vi "Measurement UI.vi"() -> ()   [LabVIEW 2025]
panel:
  in  "MeasGraphs":T1(tab)
  out "EfficiencyGraph":T2(graph)
  out "LoadRegulationGraph(V/A)":T2(graph)
  out "LoadRegulationGraph(%)":T2(graph)
  out "Load voltage deviation":dbl
  out "Load voltages":dbl
  out "Efficiency":dbl
  out "Load currents":dbl
  in  "Source Voltage":dbl=6.0 format="%#_6pV"
  in  "Load Current":dbl=5.0 format="%#_6pA"
  in  "Buffer graph":bool=TRUE
  in  "Load sense":i32(ring)=1009 caption="SENSE" items=["Local"=1008, "Remote"=1009]
  in  "Source sense":i32(ring)=1009 caption="SENSE" items=["Local"=1008, "Remote"=1009]
  out "Status":string
  in  "Load resource name":refnum<k15> caption="RESOURCE NAME"
  in  "Source resource name":refnum<k15> caption="RESOURCE NAME"
  in  "DUT setup time":dbl=1.0 caption="DUT SETUP TIME" format="%#_6ps"
  in  "Aperture time":dbl=0.005 caption="APERTURE TIME" format="%#_6ps"
  in  "Source delay":dbl=0.005 caption="SOURCE DELAY" format="%#_6ps"
  in  "Load voltage limit range":dbl=6.0 caption="VOLTAGE LIMIT RANGE" format="%#_6pV"
  in  "Source current limit":dbl=25.0 caption="CURRENT LIMIT" format="%#_6pA"
  in  "Source maximum power":dbl=140.0 caption="MAXIMUM POWER" format="%#_6pW"
  in  "Load configuration":string="Load configuration"
  in  "Source configuration":string="Source configuration"
  in  "Measurement settings":string="Measurement settings"
  in  "Nominal output voltage":dbl=3.3 caption="NOMINAL OUTPUT VOLTAGE" format="%#_6pV"
  in  "Mode of operation":T3(ring)=enum."Perform measurement" caption="MODE OF OPERATION"
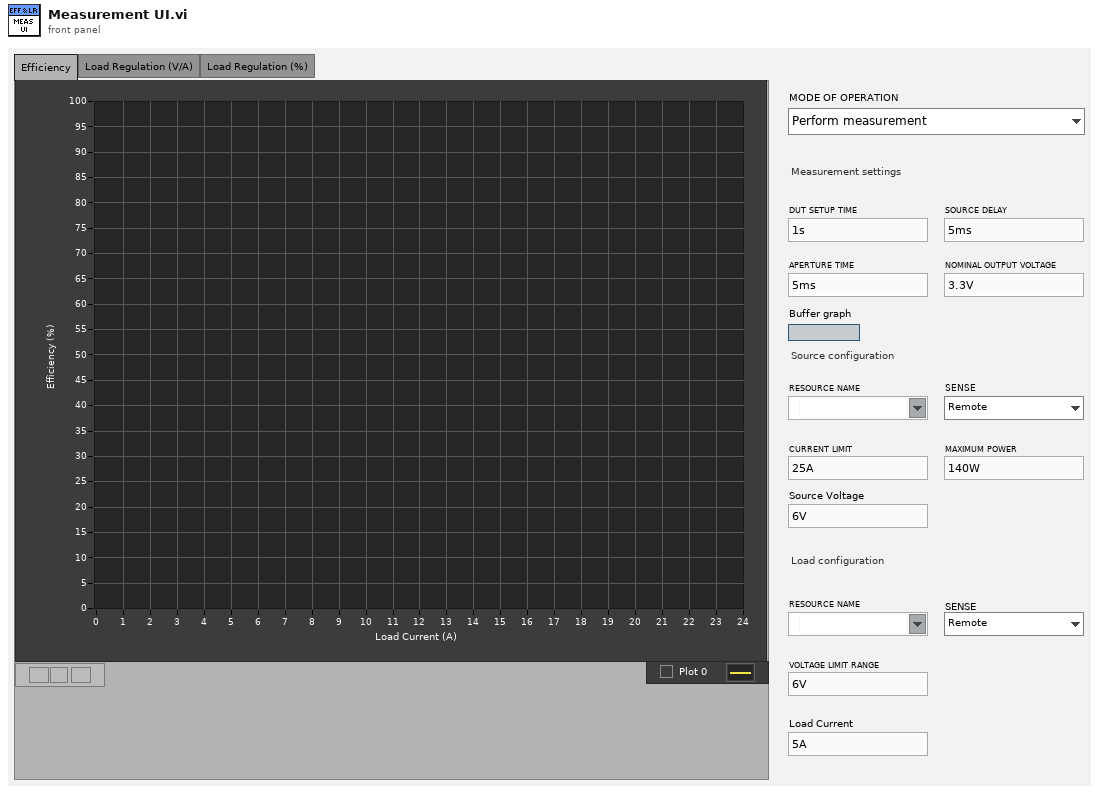
[diagram p1: front panel]
types:
  T1 = enum32{"Efficiency", "Load Regulation (V/A)", "Load Regulation (%)", "Hidden Controls"}
  T2 = cluster{"Load currents":dbl[], "Efficiency":dbl[]}[]
  T3 = enum32{"Power on the DUT", "Perform measurement", "Power off the DUT"}
  T4 = cluster{"Source Voltage[]":dbl[], "Load Current[]":dbl[], "EfficiencyGraph":cluster{"Load currents":dbl[], "Efficiency":dbl[]}[], "LoadGraph(V/A)":cluster{"Load currents":dbl[], "Efficiency":dbl[]}[], "LoadGraph(%)":cluster{"Load currents":dbl[], "Efficiency":dbl[]}[], "Execution Time":timestamp, "Debug file":path}
  T5 = cluster{"Load currents":dbl[], "Efficiency":dbl[]}
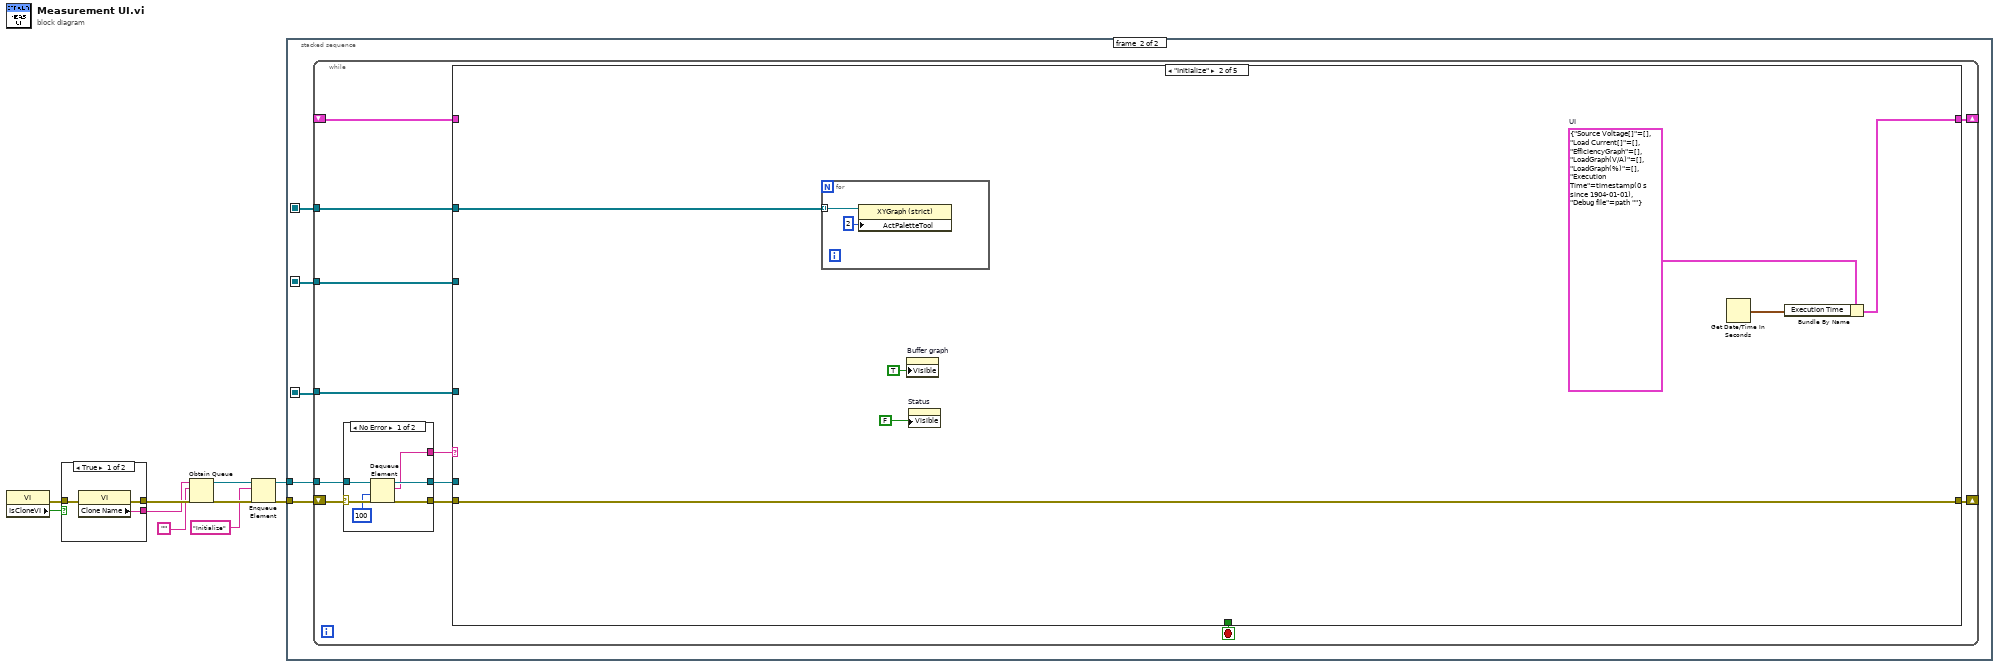
[diagram p0: block diagram]
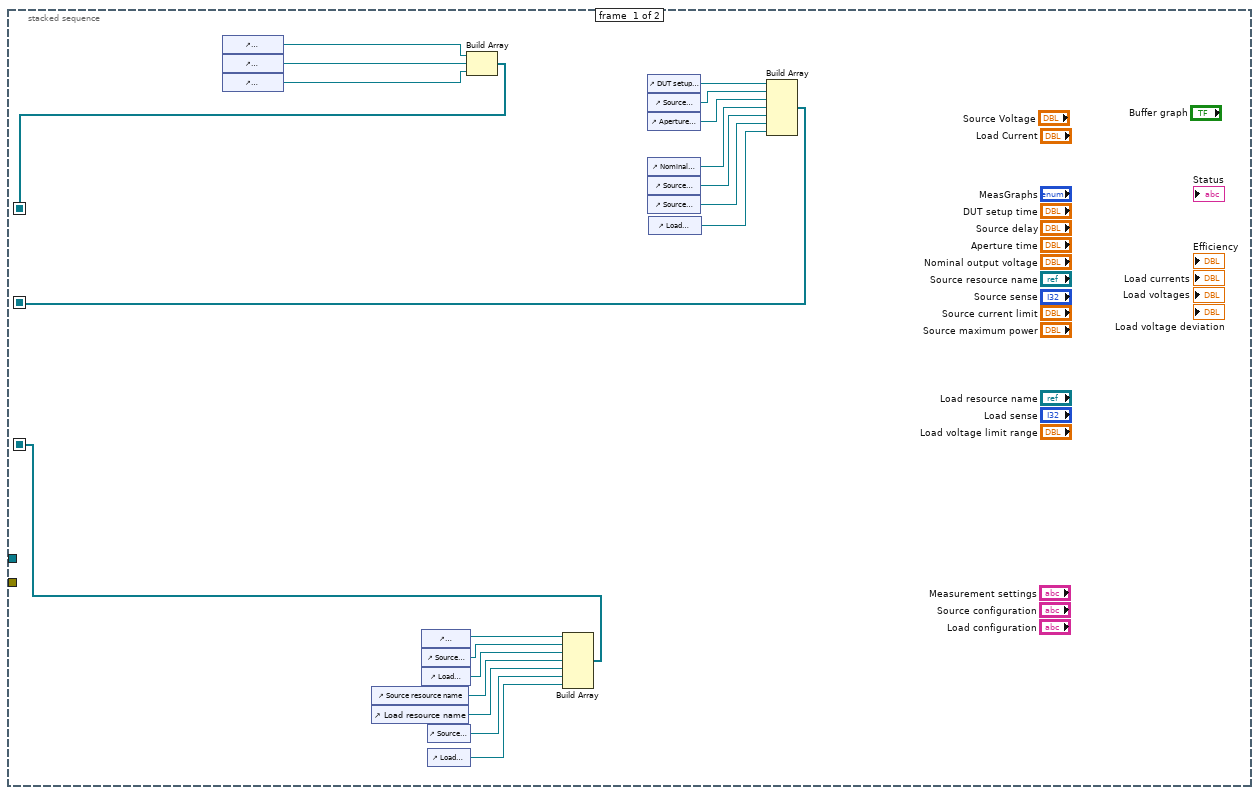
[diagram p2: hidden frame]
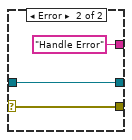
[diagram p3: hidden frame]
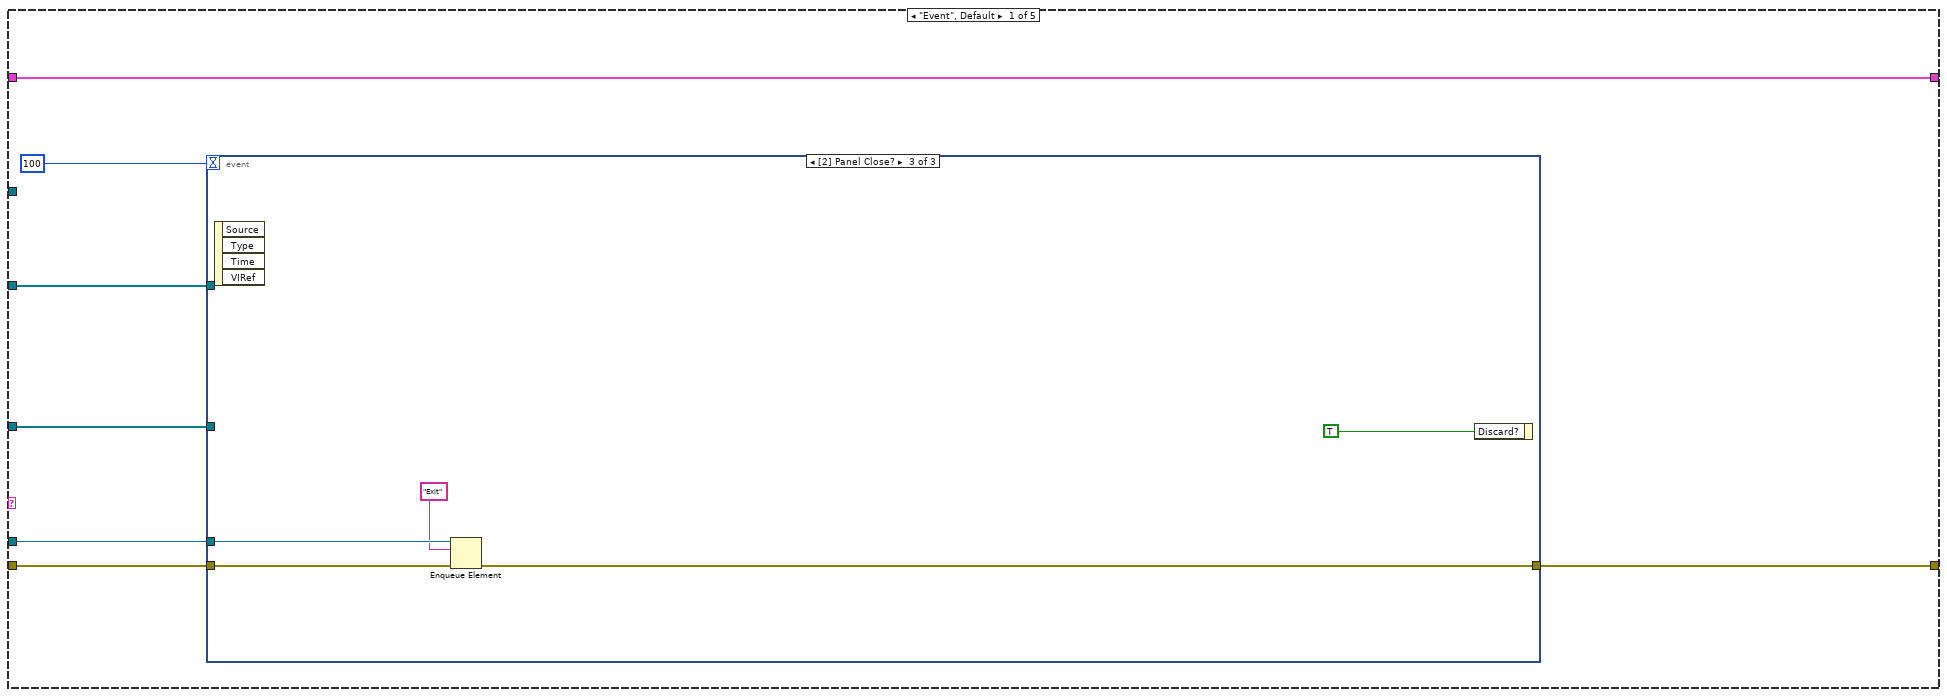
[diagram p4: hidden frame]
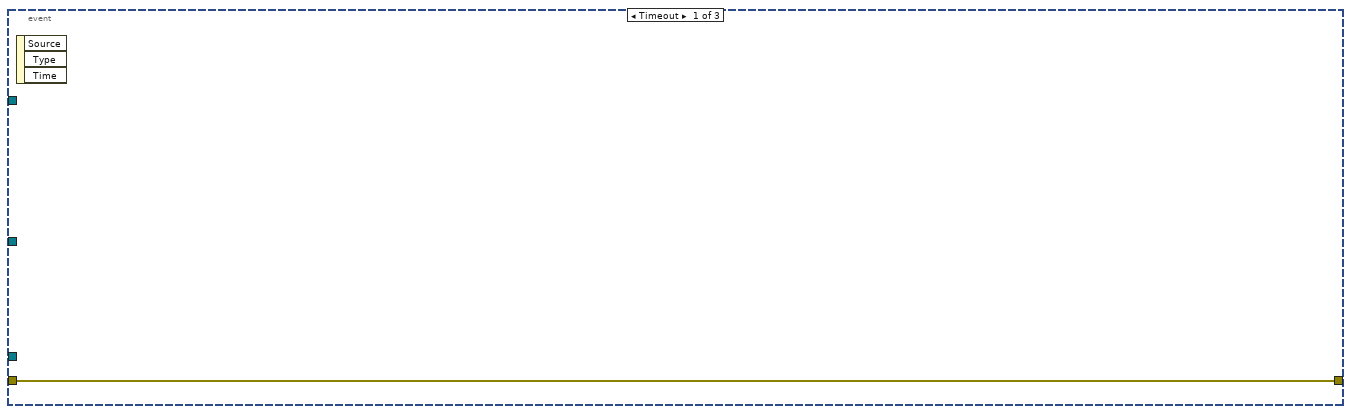
[diagram p5: hidden frame]
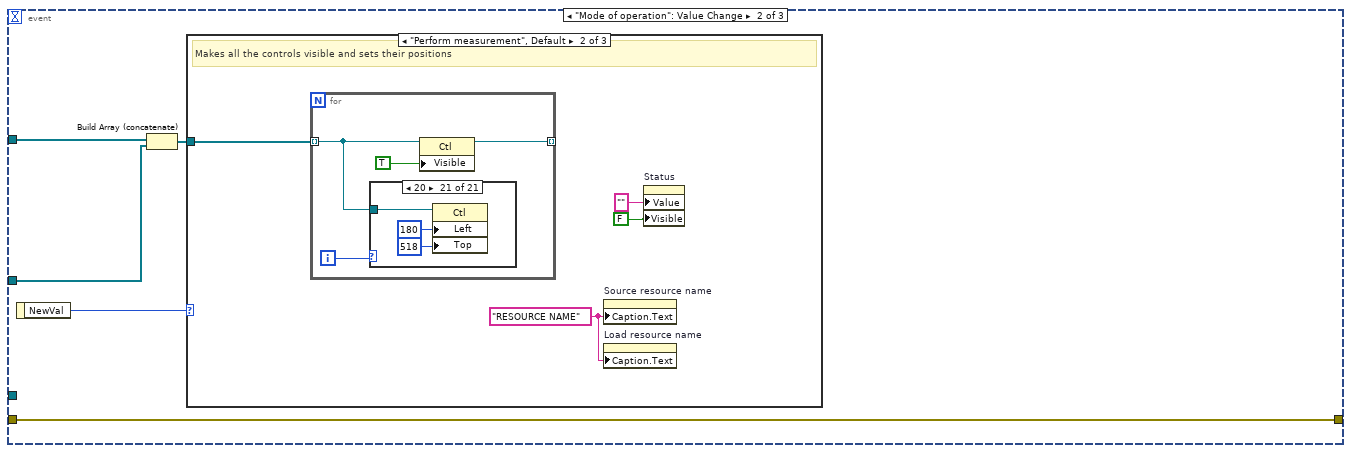
[diagram p6: hidden frame]
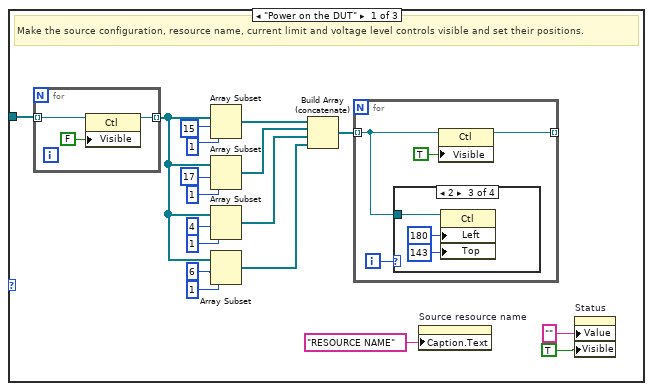
[diagram p7: hidden frame]
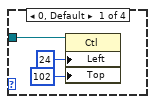
[diagram p8: hidden frame]
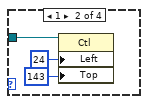
[diagram p9: hidden frame]
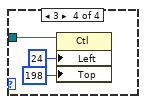
[diagram p10: hidden frame]
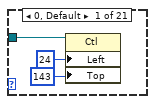
[diagram p11: hidden frame]
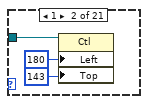
[diagram p12: hidden frame]
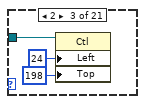
[diagram p13: hidden frame]
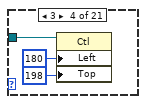
[diagram p14: hidden frame]
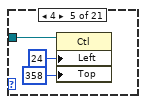
[diagram p15: hidden frame]
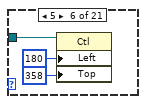
[diagram p16: hidden frame]
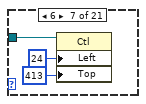
[diagram p17: hidden frame]
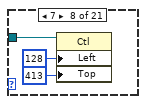
[diagram p18: hidden frame]
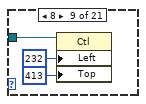
[diagram p19: hidden frame]
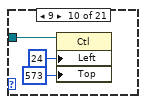
[diagram p20: hidden frame]
diagram:
  n1 = property class="VI"() -> (error out=w1:errorcluster, "IsCloneVI"=w2:bool)  [unwired: 2 in, 1 out]
  n2 = case shown="True" w2 {
    tunnel: [w13 w16] -> w10
    tunnel: [w12 w15] -> w9
    tunnel: w1 -> [w11 w14]
    frame True {
      n3 = property class="VI"(error in=w11) -> (error out=w13:errorcluster, "Clone Name"=w12:string)  [unwired: 1 in, 1 out]
    }
    frame False {
      n4 = property class="VI"(error in=w14) -> (error out=w16:errorcluster, "Name"=w15:string)  [unwired: 1 in, 1 out]
    }
  }
  n5 = Obtain Queue(name (unnamed)=w9, element data type="", error in (no error)=w10) -> (queue out=w6:refnum<queue>, error out=w8:errorcluster)  [unwired: 2 in, 1 out]
  n6 = Enqueue Element(queue=w6, element="Initialize", error in (no error)=w8) -> (queue out=w5:refnum<queue>, error out=w7:errorcluster)  [unwired: 1 in, 1 out]
  n7 = stacked-sequence {
    seq-local: [w19 _] -> [_ w39]
    seq-local: [w20 _] -> [_ w38]
    seq-local: [w21 _] -> [_ w37]
    tunnel: w7 -> [_ w41]
    tunnel: w5 -> [_ w40]
    frame #0 {
      n8 = control-ref of="EfficiencyGraph"() -> (w24:refnum<vi>)
      n9 = control-ref of="LoadRegulationGraph(V/A)"() -> (w23:refnum<vi>)
      n10 = control-ref of="LoadRegulationGraph(%)"() -> (w22:refnum<vi>)
      n11 = control-ref of="Source resource name"() -> (w26:refnum<vi>)
      n12 = control-ref of="Load resource name"() -> (w25:refnum<vi>)
      n13 = control-ref of="Measurement settings"() -> (w29:refnum<vi>)
      n14 = control-ref of="Source configuration"() -> (w27:refnum<vi>)
      n15 = control-ref of="Load configuration"() -> (w28:refnum<vi>)
      n16 = control-ref of="Source sense"() -> (w18:refnum<vi>)
      n17 = control-ref of="Load sense"() -> (w17:refnum<vi>)
      n18 = Build Array(w24, w23, w22) -> (w19:refnum<vi>[])
      n19 = Build Array(w29, w27, w28, w26, w25, w18, w17) -> (w21:refnum<vi>[])
      n20 = control-ref of="DUT setup time"() -> (w36:refnum<vi>)
      n21 = control-ref of="Source delay"() -> (w35:refnum<vi>)
      n22 = control-ref of="Aperture time"() -> (w34:refnum<vi>)
      n23 = control-ref of="Nominal output voltage"() -> (w30:refnum<vi>)
      n24 = control-ref of="Source current limit"() -> (w33:refnum<vi>)
      n25 = control-ref of="Source maximum power"() -> (w32:refnum<vi>)
      n26 = control-ref of="Load voltage limit range"() -> (w31:refnum<vi>)
      n27 = Build Array(w36, w35, w34, w30, w33, w32, w31) -> (w20:refnum<vi>[])
    }
    frame #1 {
      n28 = while {
        shift-right: [w48] -> _
        shift-left: w41 -> [w53]
        tunnel: w40 -> [w51]
        tunnel: w38 -> [w46]
        tunnel: w37 -> [w45]
        tunnel: w39 -> [w44]
        shift-right: [w43] -> _
        shift-left: _ -> [w42]
        stop <- w47 stop-if-true
        n29 = case shown="No Error" w53 {
          selector: w53 -> [w59 w62]
          tunnel: [w58 w62] -> w52
          tunnel: w51 -> [w57 w61]
          tunnel: [w56 w61] -> w50
          tunnel: [w55 "Handle Error"] -> w49
          frame No Error {
            n30 = Dequeue Element(queue=w57, timeout in ms (-1)=100, error in (no error)=w59) -> (queue out=w56:refnum<queue>, element=w55:string, error out=w58:errorcluster)  [unwired: 1 out]
          }
          frame Error {
          }
        }
        n31 = case shown="\"Initialize\"" w49 {
          tunnel: w52 -> [w68 w211 w222 w382 w384]
          tunnel: w50 -> [w66 _ w221 w380 _]
          tunnel: [w69 w211 w220 w374 w384] -> w48
          tunnel: [_ _ _ TRUE _] -> w47
          tunnel: w46 -> [w65 _ _ w372 _]
          tunnel: w45 -> [w64 _ _ w371 _]
          tunnel: w44 -> [_ w217 w230 w373 _]
          tunnel: [w63 w214 w229 w369 w383] -> w43
          tunnel: w42 -> [w63 _ w228 w369 w383]
          frame "Event", Default {
            n32 = event shown="[2] Panel Close?" {
              selector: _ -> [_ _ _]
              dyn-events: _ -> [_ _ _]
              timeout: 100 -> [_ _ _]
              tunnel: [w70 w71 w208] -> w69
              tunnel: w68 -> [w70 w71 w209]
              tunnel: w66 -> [_ _ w207]
              tunnel: w65 -> [_ w72 _]
              tunnel: w64 -> [_ w74 _]
              event Timeout {
                n33 = event-data() -> ()  [unwired: 1 in, 3 out]
              }
              event "Mode of operation": Value Change {
                n34 = event-data() -> ("NewVal"=w75:T3)  [unwired: 1 in]
                n35 = Build Array (concatenate)(w72, w74) -> (w73:refnum<vi>[])
                n36 = case shown="\"Perform measurement\", Default" w75 {
                  tunnel: w73 -> [w85 w116 w189]
                  frame "Power on the DUT" {
                    # "Make the source configuration, resource name, current limit and voltage level controls visible and set their positions."
                    n37 = for {
                      tunnel: w85 -> [w96] mode=indexing
                      tunnel: [w94] -> w82 mode=indexing
                      n38 = property class="Ctl"(reference=w96, "Visible"=FALSE) -> (reference out=w94:refnum<vi>)  [unwired: 1 in, 1 out]
                    }
                    n39 = Array Subset(array=w82, index=15 ("length"), length=1 ("index")) -> (w84:refnum<vi>[])
                    n40 = Array Subset(array=w82, index=17 ("length"), length=1 ("index")) -> (w83:refnum<vi>[])
                    n41 = Array Subset(array=w82, index=4 ("length"), length=1 ("index")) -> (w81:refnum<vi>[])
                    n42 = Array Subset(array=w82, index=6 ("length"), length=1 ("index")) -> (w79:refnum<vi>[])
                    n43 = Build Array (concatenate)(w84, w83, w81, w79) -> (w80:refnum<vi>[])
                    n44 = for {
                      tunnel: [w99] -> _ mode=indexing
                      tunnel: w80 -> [w97] mode=indexing
                      i -> [w98]
                      n45 = case shown="2" w98 {
                        tunnel: w97 -> [w103 w106 w109 w112]
                        frame 0, Default {
                          n46 = property class="Ctl"(reference=w103, "Left"=24 ("Position:Left"), "Top"=102 ("Position:Top")) -> ()  [unwired: 1 in, 2 out]
                        }
                        frame 1 {
                          n47 = property class="Ctl"(reference=w106, "Left"=24 ("Position:Left"), "Top"=143 ("Position:Top")) -> ()  [unwired: 1 in, 2 out]
                        }
                        frame 2 {
                          n48 = property class="Ctl"(reference=w109, "Left"=180 ("Position:Left"), "Top"=143 ("Position:Top")) -> ()  [unwired: 1 in, 2 out]
                        }
                        frame 3 {
                          n49 = property class="Ctl"(reference=w112, "Left"=24 ("Position:Left"), "Top"=198 ("Position:Top")) -> ()  [unwired: 1 in, 2 out]
                        }
                      }
                      n50 = property class="Ctl"(reference=w97, "Visible"=TRUE) -> (reference out=w99:refnum<vi>)  [unwired: 1 in, 1 out]
                    }
                    n51 = property on="Source resource name" class="IVIName"("Caption.Text"="RESOURCE NAME") -> ()  [unwired: 2 in, 2 out]
                    n52 = property on="Status" class="Str"("Value"="" ("Status"), "Visible"=TRUE) -> ()  [unwired: 2 in, 2 out]
                  }
                  frame "Perform measurement", Default {
                    w115 = "RESOURCE NAME" ("Caption.Text")
                    # "Makes all the controls visible and sets their positions"
                    n53 = for {
                      tunnel: w116 -> [w117] mode=indexing
                      tunnel: [w119] -> _ mode=indexing
                      i -> [w118]
                      n54 = case shown="20" w118 {
                        tunnel: w117 -> [w123 w126 w129 w132 w135 w138 w141 w144 w147 w150 w153 w156 w159 w162 w165 w168 w171 w174 w177 w178 w181]
                        frame 0, Default {
                          n55 = property class="Ctl"(reference=w123, "Left"=24 ("Position:Left"), "Top"=143 ("Position:Top")) -> ()  [unwired: 1 in, 2 out]
                        }
                        frame 1 {
                          n56 = property class="Ctl"(reference=w126, "Left"=180 ("Position:Left"), "Top"=143 ("Position:Top")) -> ()  [unwired: 1 in, 2 out]
                        }
                        frame 2 {
                          n57 = property class="Ctl"(reference=w129, "Left"=24 ("Position:Left"), "Top"=198 ("Position:Top")) -> ()  [unwired: 1 in, 2 out]
                        }
                        frame 3 {
                          n58 = property class="Ctl"(reference=w132, "Left"=180 ("Position:Left"), "Top"=198 ("Position:Top")) -> ()  [unwired: 1 in, 2 out]
                        }
                        frame 4 {
                          n59 = property class="Ctl"(reference=w135, "Left"=24 ("Position:Left"), "Top"=358 ("Position:Top")) -> ()  [unwired: 1 in, 2 out]
                        }
                        frame 5 {
                          n60 = property class="Ctl"(reference=w138, "Left"=180 ("Position:Left"), "Top"=358 ("Position:Top")) -> ()  [unwired: 1 in, 2 out]
                        }
                        frame 6 {
                          n61 = property class="Ctl"(reference=w141, "Left"=24 ("Position:Left"), "Top"=413 ("Position:Top")) -> ()  [unwired: 1 in, 2 out]
                        }
                        frame 7 {
                          n62 = property class="Ctl"(reference=w144, "Left"=128 ("Position:Left"), "Top"=413 ("Position:Top")) -> ()  [unwired: 1 in, 2 out]
                        }
                        frame 8 {
                          n63 = property class="Ctl"(reference=w147, "Left"=232 ("Position:Left"), "Top"=413 ("Position:Top")) -> ()  [unwired: 1 in, 2 out]
                        }
                        frame 9 {
                          n64 = property class="Ctl"(reference=w150, "Left"=24 ("Position:Left"), "Top"=573 ("Position:Top")) -> ()  [unwired: 1 in, 2 out]
                        }
                        frame 10 {
                          n65 = property class="Ctl"(reference=w153, "Left"=180 ("Position:Left"), "Top"=573 ("Position:Top")) -> ()  [unwired: 1 in, 2 out]
                        }
                        frame 11 {
                          n66 = property class="Ctl"(reference=w156, "Left"=24 ("Position:Left"), "Top"=628 ("Position:Top")) -> ()  [unwired: 1 in, 2 out]
                        }
                        frame 12 {
                          n67 = property class="Ctl"(reference=w159, "Left"=128 ("Position:Left"), "Top"=628 ("Position:Top")) -> ()  [unwired: 1 in, 2 out]
                        }
                        frame 13 {
                          n68 = property class="Ctl"(reference=w162, "Left"=232 ("Position:Left"), "Top"=628 ("Position:Top")) -> ()  [unwired: 1 in, 2 out]
                        }
                        frame 14 {
                          n69 = property class="Ctl"(reference=w165, "Left"=24 ("Position:Left"), "Top"=102 ("Position:Top")) -> ()  [unwired: 1 in, 2 out]
                        }
                        frame 15 {
                          n70 = property class="Ctl"(reference=w168, "Left"=24 ("Position:Left"), "Top"=262 ("Position:Top")) -> ()  [unwired: 1 in, 2 out]
                        }
                        frame 16 {
                          n71 = property class="Ctl"(reference=w171, "Left"=24 ("Position:Left"), "Top"=477 ("Position:Top")) -> ()  [unwired: 1 in, 2 out]
                        }
                        frame 17 {
                          n72 = property class="Ctl"(reference=w174, "Left"=24 ("Position:Left"), "Top"=303 ("Position:Top")) -> ()  [unwired: 1 in, 2 out]
                        }
                        frame 18 {
                          n73 = property class="Ctl"(reference=w177, "Left"=24 ("Position:Left"), "Top"=518 ("Position:Top")) -> ()  [unwired: 1 in, 2 out]
                        }
                        frame 19 {
                          n74 = property class="Ctl"(reference=w178, "Left"=180 ("Position:Left"), "Top"=303 ("Position:Top")) -> ()  [unwired: 1 in, 2 out]
                        }
                        frame 20 {
                          n75 = property class="Ctl"(reference=w181, "Left"=180 ("Position:Left"), "Top"=518 ("Position:Top")) -> ()  [unwired: 1 in, 2 out]
                        }
                      }
                      n76 = property class="Ctl"(reference=w117, "Visible"=TRUE) -> (reference out=w119:refnum<vi>)  [unwired: 1 in, 1 out]
                    }
                    n77 = property on="Source resource name" class="IVIName"("Caption.Text"=w115) -> ()  [unwired: 2 in, 2 out]
                    n78 = property on="Load resource name" class="IVIName"("Caption.Text"=w115) -> ()  [unwired: 2 in, 2 out]
                    n79 = property on="Status" class="Str"("Value"="" ("Status"), "Visible"=FALSE) -> ()  [unwired: 2 in, 2 out]
                  }
                  frame "Power off the DUT" {
                    # "Makes only the Source and Load Resource Name controls visible and sets their positions"
                    n80 = for {
                      tunnel: w189 -> [w194] mode=indexing
                      tunnel: [w193] -> w188 mode=indexing
                      n81 = property class="Ctl"(reference=w194, "Visible"=FALSE) -> (reference out=w193:refnum<vi>)  [unwired: 1 in, 1 out]
                    }
                    n82 = Array Subset(array=w188, index=17 ("length"), length=2 ("index")) -> (w190:refnum<vi>[])
                    n83 = property on="Source resource name" class="IVIName"("Caption.Text"="SOURCE RESOURCE NAME") -> ()  [unwired: 2 in, 2 out]
                    n84 = property on="Load resource name" class="IVIName"("Caption.Text"="LOAD RESOURCE NAME") -> ()  [unwired: 2 in, 2 out]
                    n85 = for {
                      tunnel: w190 -> [w196] mode=indexing
                      tunnel: [w198] -> _ mode=indexing
                      i -> [w197]
                      n86 = case shown="0, Default" w197 {
                        tunnel: w196 -> [w202 w205]
                        frame 0, Default {
                          n87 = property class="Ctl"(reference=w202, "Left"=24 ("Position:Left"), "Top"=102 ("Position:Top")) -> ()  [unwired: 1 in, 2 out]
                        }
                        frame 1 {
                          n88 = property class="Ctl"(reference=w205, "Left"=24 ("Position:Left"), "Top"=157 ("Position:Top")) -> ()  [unwired: 1 in, 2 out]
                        }
                      }
                      n89 = property class="Ctl"(reference=w196, "Visible"=TRUE) -> (reference out=w198:refnum<vi>)  [unwired: 1 in, 1 out]
                    }
                    n90 = property on="Status" class="Str"("Value"="" ("Status"), "Visible"=TRUE) -> ()  [unwired: 2 in, 2 out]
                  }
                }
              }
              event Panel Close? {
                n91 = event-data() -> ()  [unwired: 1 in, 4 out]
                n92 = Enqueue Element(queue=w207, element="Exit", error in (no error)=w209) -> (error out=w208:errorcluster)  [unwired: 1 in, 2 out]
                n93 = event-data("Discard?"=TRUE) -> ()  [unwired: 1 in, 1 out]
              }
            }
          }
          frame "Initialize" {
            w215 = T4 {"Source Voltage[]"=[], "Load Current[]"=[], "EfficiencyGraph"=[], "LoadGraph(V/A)"=[], "LoadGraph(%)"=[], "Execution Time"=timestamp(0 s since 1904-01-01), "Debug file"=path ""}  # UI
            n94 = for {
              tunnel: w217 -> [w218] mode=indexing
              n95 = property class="XYGraph (strict)"(reference=w218, "ActPaletteTool"=2 ("Palette:Active Tool")) -> ()  [unwired: 1 in, 2 out]
            }
            n96 = property on="Buffer graph" class="Bool (strict)"("Visible"=TRUE) -> ()  [unwired: 2 in, 2 out]
            n97 = property on="Status" class="Str"("Visible"=FALSE) -> ()  [unwired: 2 in, 2 out]
            n98 = Get Date/Time In Seconds() -> (seconds since 1Jan1904=w212:timestamp)
            n99 = Bundle By Name(cluster=w215, "Execution Time"=w212) -> (w214:T4)
          }
          frame "Post UI Update" {
            w224 = 5.0  # reset in sec
            # "This case will be triggered, after framework updates the User interface with result values."
            n100 = Unbundle By Name(w228) -> ("Execution Time"=w226:timestamp)
            n101 = Get Date/Time In Seconds() -> (seconds since 1Jan1904=w227:timestamp)
            n102 = Subtract(x=w227, y=w226) -> (x-y=w225:dbl)
            n103 = Less?(x=w225, y=w224) -> (x < y?=w223:bool)
            n104 = case shown="False" w223 {
              tunnel: w230 -> [_ w258]
              tunnel: w228 -> [w233 w251]
              tunnel: [w232 w245] -> w229
              tunnel: w222 -> [w236 w246]
              tunnel: w221 -> [w235 _]
              tunnel: [w234 w246] -> w220
              frame False {
                # "Assuming that the user will take atleast 5 seconds for next sequence run.\nThe 5 seconds value chosed because measurement always took more than\n5 seconds to execute."
                n105 = disable-structure shown="Enabled" {
                  disable-tunnel: w236 -> [w241 w242]
                  disable-tunnel: w235 -> [w240 _]
                  disable-tunnel: [w237 w242] -> w234
                  frame Enabled {
                    n106 = Enqueue Element(queue=w240, element="Initialize", timeout in ms (-1)=100, error in (no error)=w241) -> (error out=w237:errorcluster)  [unwired: 2 out]
                  }
                  frame Disabled {
                  }
                }
                n107 = Get Date/Time In Seconds() -> (seconds since 1Jan1904=w231:timestamp)
                n108 = Bundle By Name(cluster=w233, "Execution Time"=w231) -> (w232:T4)
              }
              frame True {
                w247 = u32[] [15787074, 5682409, 15535092, 40563, 13983232, 35009, 15113984, 13400487, 15993633, 10221451, 8148942, 15869817, 32914, 10196480, 6271923, 16355671]  # Plot colors
                # "-Sets various properties of graphs like color, point style, plot name etc.\n-Increases the legend number of rows if the voltage values are less than 4 and \nif it is greater than 4 then make the default rows as 4 and enable the vertical scrollbar.\n-Also sets the plot minimum property to source sweep points which disables the unused plots in the graph."
                n109 = Unbundle By Name(w251) -> ("Source Voltage[]"=w252:dbl[])
                n110 = for {
                  tunnel: w252 -> [w353]
                  tunnel: w258 -> [w352] mode=indexing
                  tunnel: w247 -> [w351]
                  n111 = for {
                    tunnel: w353 -> [w365] mode=indexing
                    tunnel: w352 -> [w360]
                    tunnel: w351 -> [w363] mode=indexing
                    i -> [w361]
                    n112 = Increment(x=w361) -> (x+1=w359:i32)
                    n113 = To Unsigned Long Integer(number=w361) -> (unsigned 32bit integer=w364:u32)
                    n114 = Format Value(format string="%.3f", value (0)=w365) -> (output string=w368:string)  [unwired: 1 out]
                    n115 = property on="Property Node" class="XYGraph (strict)"(reference=w360, "LegScrollVis"=FALSE ("Legend:Scrollbar Visible"), "LegNumRows"=w359, "LegPlotMin"=1 ("y")) -> (reference out=w358:refnum<vi>, error out=w357:errorcluster)  [unwired: 1 in]
                    n116 = Concatenate Strings(" Vin = " ("string"), w368) -> (w356:string)
                    n117 = property on="Property Node" class="XYGraph (strict)"(reference=w358, error in=w357, "Active Plot"=w364, "Plot.Point Style"=u8 5, "Plot.Plot Color"=w363, "Plot.Fill/Pt. Color"=w363, "Plot.Plot Name"=w356) -> ()  [unwired: 2 out]
                  }
                }
                n118 = local read "Load voltage deviation"() -> (w253:dbl)
                n119 = local read "Load voltages"() -> (w254:dbl)
                n120 = local read "Load currents"() -> (w256:dbl)
                n121 = local read "Buffer graph"() -> (w257:bool)
                n122 = local read "Efficiency"() -> (w255:dbl)
                n123 = case shown="True" w257 {
                  tunnel: w251 -> [w273 w279]
                  tunnel: w256 -> [w277 w285]
                  tunnel: w255 -> [w274 w291]
                  tunnel: w254 -> [w269 w288]
                  tunnel: w253 -> [w268 w284]
                  tunnel: [w275 w290] -> w243
                  tunnel: [w271 w280] -> w250
                  tunnel: [w260 w287] -> w249
                  tunnel: [w259 w283] -> w248
                  frame False {
                    w272 = T2 [] ("EfficiencyGraph")
                    w262 = T5 {"Load currents"=[], "Efficiency"=[]} ("EfficiencyGraph")
                    w267 = dbl[] [] ("Source Voltage")
                    n124 = Insert Into Array(array=w267, new element=w277) -> (w266:dbl[])  [unwired: 1 in]
                    n125 = Insert Into Array(array=w267, new element=w274) -> (w270:dbl[])  [unwired: 1 in]
                    n126 = Insert Into Array(array=w267, new element=w269) -> (w265:dbl[])  [unwired: 1 in]
                    n127 = Insert Into Array(array=w267, new element=w268) -> (w264:dbl[])  [unwired: 1 in]
                    n128 = Bundle(cluster=w262, "Load currents"=w266, "Efficiency"=w270) -> (w276:T5)
                    n129 = Bundle(cluster=w262, "Load currents"=w266, "Efficiency"=w265) -> (w263:T5)
                    n130 = Bundle(cluster=w262, "Load currents"=w266, "Efficiency"=w264) -> (w261:T5)
                    n131 = Bundle By Name(cluster=w273, "Source Voltage[]"=w267, "Load Current[]"=w267, "EfficiencyGraph"=w272, "LoadGraph(V/A)"=w272, "LoadGraph(%)"=w272) -> (w271:T4)
                    n132 = Build Array(w276) -> (w275:T2)
                    n133 = Build Array(w263) -> (w260:T2)
                    n134 = Build Array(w261) -> (w259:T2)
                  }
                  frame True {
                    n135 = Unbundle By Name(w279) -> ("Source Voltage[]"=w281:dbl[], "EfficiencyGraph"=w292:T2, "LoadGraph(V/A)"=w289:T2, "LoadGraph(%)"=w286:T2)
                    n136 = local read "Source Voltage"() -> (w278:dbl)
                    n137 = Delete From Array(array=w281) -> (deleted portion=w293:dbl)  [unwired: 2 in, 1 out]
                    n138 = Not Equal?(x=w293, y=w278) -> (x != y?=w282:bool)
                    n139 = case shown="False" w282 {
                      tunnel: w292 -> [w313 w317]
                      tunnel: w291 -> [w315 w347]
                      tunnel: [w300 w325] -> w290
                      tunnel: w289 -> [w310 w337]
                      tunnel: w288 -> [w309 w336]
                      tunnel: [w299 w324] -> w287
                      tunnel: w286 -> [w308 w328]
                      tunnel: w285 -> [w306 w320]
                      tunnel: w284 -> [w305 w327]
                      tunnel: [w298 w323] -> w283
                      tunnel: [w301 w326] -> w280
                      tunnel: w279 -> [w297 w322]
                      tunnel: w278 -> [w295 _]
                      frame True {
                        n140 = Unbundle By Name(w297) -> ("Source Voltage[]"=w296:dbl[])
                        n141 = Build Array(w306) -> (w304:dbl[])
                        n142 = Build Array(w315) -> (w314:dbl[])
                        n143 = Build Array(w309) -> (w303:dbl[])
                        n144 = Build Array(w305) -> (w302:dbl[])
                        n145 = Build Array (concatenate)(w296, w295) -> (w294:dbl[])
                        n146 = Bundle(w304, w314) -> (w312:cluster{dbl[], dbl[]})  [unwired: 1 in]
                        n147 = Bundle(w304, w303) -> (w311:cluster{dbl[], dbl[]})  [unwired: 1 in]
                        n148 = Bundle(w304, w302) -> (w307:cluster{dbl[], dbl[]})  [unwired: 1 in]
                        n149 = Insert Into Array(array=w313, new element=w312) -> (w300:T2)  [unwired: 1 in]
                        n150 = Insert Into Array(array=w310, new element=w311) -> (w299:T2)  [unwired: 1 in]
                        n151 = Insert Into Array(array=w308, new element=w307) -> (w298:T2)  [unwired: 1 in]
                        n152 = Bundle By Name(cluster=w297, "Source Voltage[]"=w294, "EfficiencyGraph"=w300, "LoadGraph(V/A)"=w299, "LoadGraph(%)"=w298) -> (w301:T4)
                      }
                      frame False {
                        n153 = Unbundle By Name(w322) -> ("Load Current[]"=w321:dbl[])
                        n154 = Delete From Array(array=w337) -> (deleted portion=w338:T5, array with subset deleted=w343:T2)  [unwired: 2 in]
                        n155 = Delete From Array(array=w328) -> (deleted portion=w335:T5, array with subset deleted=w330:T2)  [unwired: 2 in]
                        n156 = Delete From Array(array=w317) -> (deleted portion=w350:T5, array with subset deleted=w316:T2)  [unwired: 2 in]
                        n157 = Unbundle(w338) -> ("Load currents"=w339:dbl[], "Efficiency"=w340:dbl[])
                        n158 = Unbundle(w335) -> ("Load currents"=w334:dbl[], "Efficiency"=w333:dbl[])
                        n159 = Unbundle(w350) -> ("Load currents"=w349:dbl[], "Efficiency"=w348:dbl[])
                        n160 = Build Array (concatenate)(w339, w320) -> (w341:dbl[])
                        n161 = Build Array (concatenate)(w340, w336) -> (w342:dbl[])
                        n162 = Build Array (concatenate)(w334, w320) -> (w332:dbl[])
                        n163 = Build Array (concatenate)(w333, w327) -> (w331:dbl[])
                        n164 = Build Array (concatenate)(w349, w320) -> (w346:dbl[])
                        n165 = Build Array (concatenate)(w348, w347) -> (w345:dbl[])
                        n166 = Build Array (concatenate)(w321, w320) -> (w319:dbl[])
                        n167 = Bundle(w341, w342) -> (w344:cluster{dbl[], dbl[]})  [unwired: 1 in]
                        n168 = Bundle(w332, w331) -> (w329:cluster{dbl[], dbl[]})  [unwired: 1 in]
                        n169 = Bundle(w346, w345) -> (w318:cluster{dbl[], dbl[]})  [unwired: 1 in]
                        n170 = Insert Into Array(array=w343, new element=w344) -> (w324:T2)  [unwired: 1 in]
                        n171 = Insert Into Array(array=w330, new element=w329) -> (w323:T2)  [unwired: 1 in]
                        n172 = Insert Into Array(array=w316, new element=w318) -> (w325:T2)  [unwired: 1 in]
                        n173 = Bundle By Name(cluster=w322, "Load Current[]"=w319, "EfficiencyGraph"=w325, "LoadGraph(V/A)"=w324, "LoadGraph(%)"=w323) -> (w326:T4)
                      }
                    }
                  }
                }
                "EfficiencyGraph" <- w243
                "LoadRegulationGraph(V/A)" <- w249
                "LoadRegulationGraph(%)" <- w248
                n174 = Get Date/Time In Seconds() -> (seconds since 1Jan1904=w244:timestamp)
                n175 = Bundle By Name(cluster=w250, "Execution Time"=w244) -> (w245:T4)
              }
            }
          }
          frame "Exit" {
            # "This case is triggered to close the User Interface from framework"
            n176 = Build Array (concatenate)(w373, w372, w371) -> (w370:refnum<vi>[])
            n177 = Close Reference(reference=w370) -> (error out=w376:errorcluster)  [unwired: 1 in]
            n178 = Flush Queue(queue=w380, error in (no error)=w382) -> (queue out=w379:refnum<queue>, error out=w378:errorcluster)  [unwired: 1 out]
            n179 = Release Queue(queue=w379, force destroy? (F)=TRUE, error in (no error)=w378) -> (error out=w375:errorcluster)  [unwired: 2 out]
            n180 = Merge Errors(w376, w375) -> (w374:errorcluster)
          }
          frame "Handle Error" {
          }
        }
      }
    }
  }
